vi "List Packages.vi"() -> ()   [LabVIEW 2020]
uses:
  API Server.ctl
  Package/Get Name.vi
  Package/Get Icon.vi
  GCentral API/GCentral API.lvclass
  GCentral-API.lvlib
  Package/Package.lvclass
panel:
  out "Array":T1(array[cluster])
  out "error out":errorcluster
  in  "API Server":T2=enum."test"
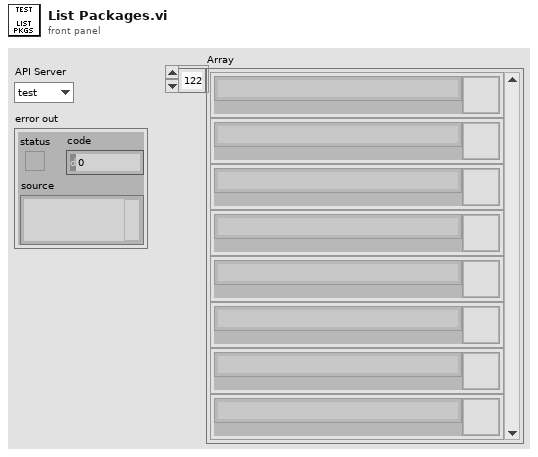
[diagram p1: front panel]
types:
  T1 = cluster{"Properties:Name":string, "Properties:Icon":picture}[]
  T2 = typedef "GCentral-API.lvlib/API Server.ctl" = enum16{"auto", "live", "test", "local"}
  T3 = cluster{"Properties:Name":string, "Properties:Icon":picture}
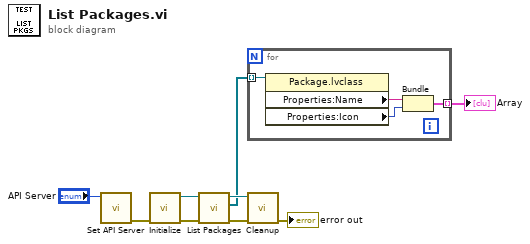
[diagram p0: block diagram]
diagram:
  n1 = call "Set API Server.vi"("API Server"="API Server") -> ("error out"=w2:errorcluster)  [unwired: 10 in]
  n2 = call "Initialize.vi"("error in (no error)"=w2) -> ("error out"=w8:errorcluster, "GCentral API out"=w9:refnum<class "GCentral API.lvclass">)  [unwired: 9 in]
  n3 = call "List Packages.vi"("error in (no error)"=w8, "GCentral API in"=w9) -> ("error out"=w6:errorcluster, "Packages"=w4:refnum<class "Package.lvclass">[], "GCentral API out"=w7:refnum<class "GCentral API.lvclass">)  [unwired: 6 in, 1 out]
  n4 = for {
    tunnel: w4 -> [w13] mode=indexing
    tunnel: [w10] -> w1 mode=indexing
    n5 = property class="Package.lvclass"(reference=w13) -> ("Properties:Name"=w12:string, "Properties:Icon"=w11:picture)  [unwired: 1 in, 2 out]
    n6 = Bundle("Properties:Name"=w12, "Properties:Icon"=w11) -> (w10:T3)  [unwired: 1 in]
  }
  "Array" <- w1
  n7 = call "Cleanup.vi"("error in (no error)"=w6, "GCentral API in"=w7) -> ("error out"=→"error out":errorcluster)  [unwired: 9 in]
